vi "fgv_userEvent.vi"(7 "Option":T1(ring)=enum."Destroy", 8 "Error In":errorcluster) -> (0 "Error Out":errorcluster, 3 "Event Registration Refnum":refnum<event-registration>)   [LabVIEW 2018, in "UI.lvclass"]
uses:
  UI.lvclass
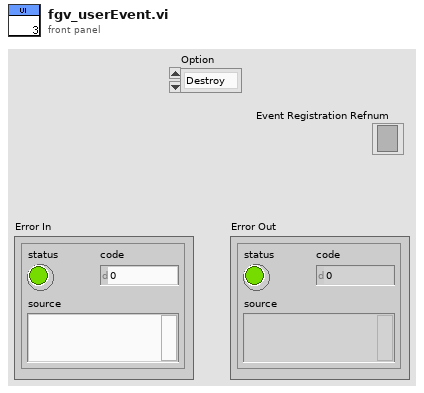
[diagram p1: front panel]
types:
  T1 = enum16{"Create", "Register", "Generate", "Unregister", "Destroy"}
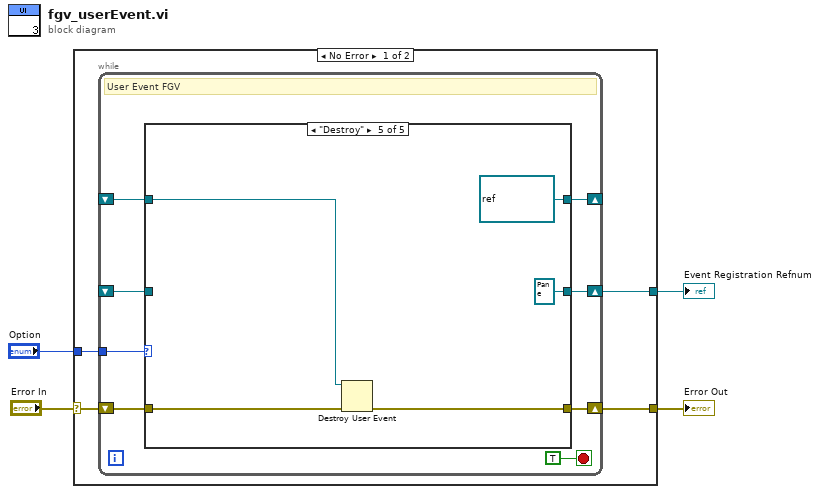
[diagram p0: block diagram]
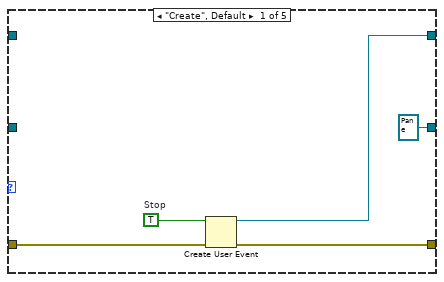
[diagram p2: hidden frame]
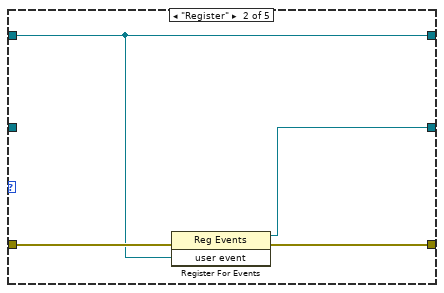
[diagram p3: hidden frame]
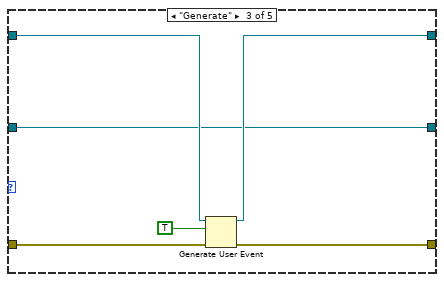
[diagram p4: hidden frame]
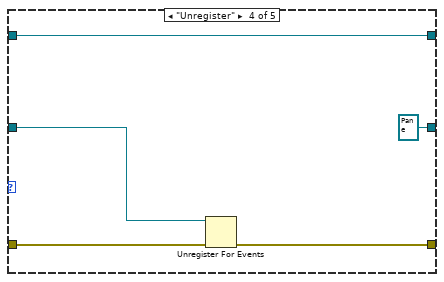
[diagram p5: hidden frame]
diagram:
  n1 = case shown="No Error" "Error In" {
    selector: "Error In" -> [w7 w42]
    tunnel: "Option" -> [w8 _]
    tunnel: [w6 w42] -> w3
    tunnel: [w5 _] -> w1
    frame No Error {
      n2 = while {
        tunnel: w8 -> [w16]
        shift-right: [w14] -> w6
        shift-left: w7 -> [w15]
        shift-right: [w13] -> _
        shift-left: _ -> [w12]
        shift-right: [w11] -> w5
        shift-left: _ -> [w10]
        stop <- TRUE stop-if-true
        # "User Event FGV"
        n3 = case shown="\"Destroy\"" w16 {
          tunnel: w15 -> [w21 w25 w31 w36 w41]
          tunnel: [w20 w24 w30 w35 w40] -> w14
          tunnel: [w19 w22 w28 w33 refnum<user-event> refnum ("user event")] -> w13
          tunnel: w12 -> [_ w22 w29 w33 w39]
          tunnel: [refnum<event-registration> refnum ("Event Registration Refnum") w23 w26 refnum<event-registration> refnum ("Event Registration Refnum") refnum<event-registration> refnum ("Event Registration Refnum")] -> w11
          tunnel: w10 -> [_ _ w26 w34 _]
          frame "Create", Default {
            w18 = TRUE  # Stop
            n4 = Create User Event(user event datatype=w18, error in=w21) -> (user event=w19:refnum<user-event>, error out=w20:errorcluster)
          }
          frame "Register" {
            n5 = register-events(error in=w25, w22) -> (reference out=w23:refnum<event-registration>, error out=w24:errorcluster)  [unwired: 1 in]
          }
          frame "Generate" {
            n6 = Generate User Event(user event=w29, event data cluster=TRUE ("event data"), error in=w31) -> (user event out=w28:refnum<user-event>, error out=w30:errorcluster)  [unwired: 1 in]
          }
          frame "Unregister" {
            n7 = Unregister For Events(event registration refnum=w34, error in=w36) -> (error out=w35:errorcluster)
          }
          frame "Destroy" {
            n8 = Destroy User Event(user event=w39, error in=w41) -> (error out=w40:errorcluster)
          }
        }
      }
    }
    frame Error {
    }
  }
  "Error Out" <- w3
  "Event Registration Refnum" <- w1
